vi "Get Description.vi"(11 "Beverage in":refnum<class "Beverage.lvclass">) -> (2 "Description":string, 3 "Beverage out":refnum<class "Beverage.lvclass">)   [LabVIEW 2011, in "Beverage.lvclass"]
uses:
  Beverage.lvclass
  Beverage.lvclass/Beverage.ctl
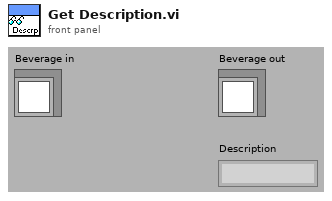
[diagram p1: front panel]
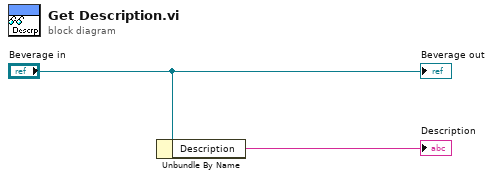
[diagram p0: block diagram]
diagram:
  n1 = Unbundle By Name("Beverage in") -> ("Description"=→"Description":string)
  "Beverage out" <- "Beverage in"
